vi "AA TCP Send Image.vi"(0 "Connection ID":refnum<k5>, 2 "Spooler Code":u8, 7 "Image Stack (U16)":u16[][][](array[numeric]), 11 "Error In":errorcluster, 13 "Setup Name":string) -> (4 "Connection ID Out":refnum<k5>, 8 "Success?":bool, 15 "Error Out":errorcluster)   [LabVIEW 2020]
panel:
  out "Image Size":i32[](array[numeric])
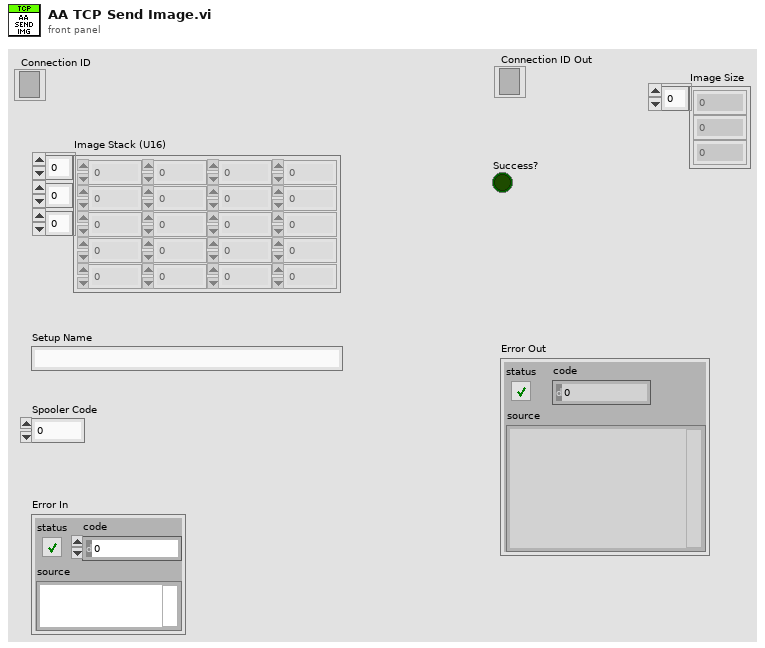
[diagram p1: front panel]
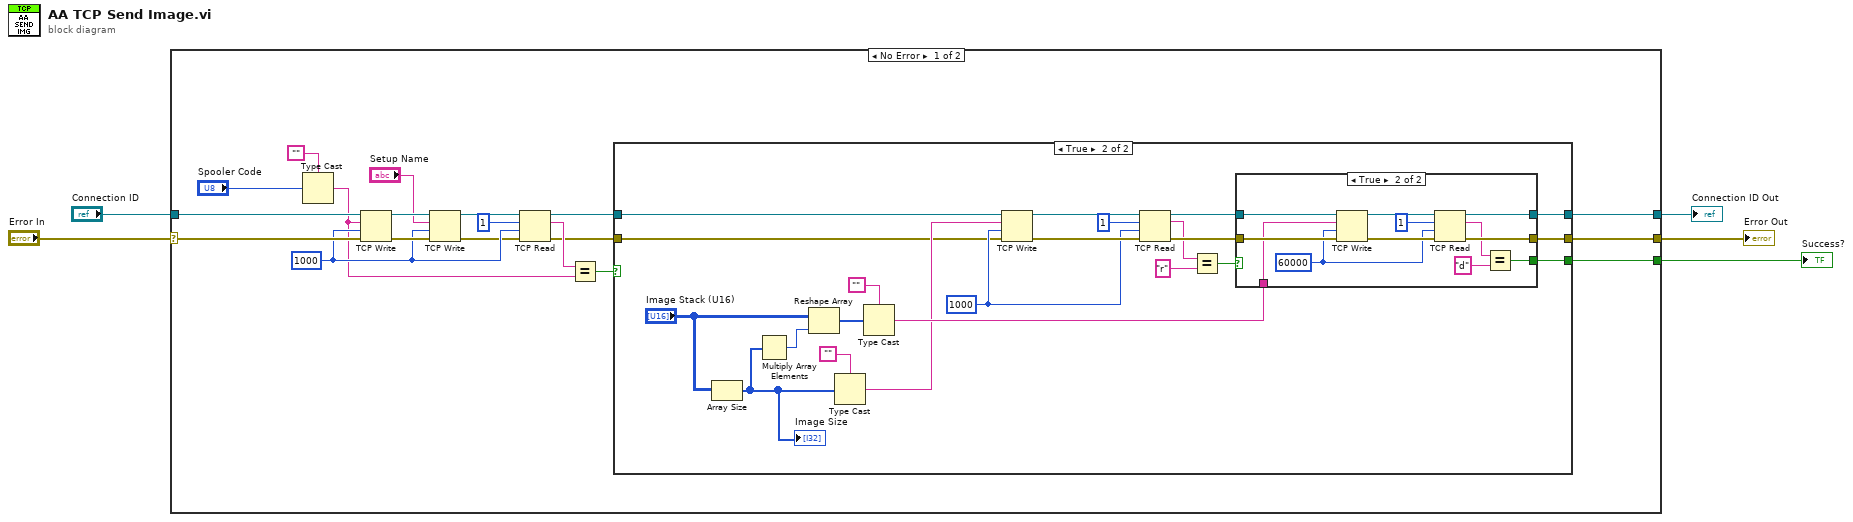
[diagram p0: block diagram]
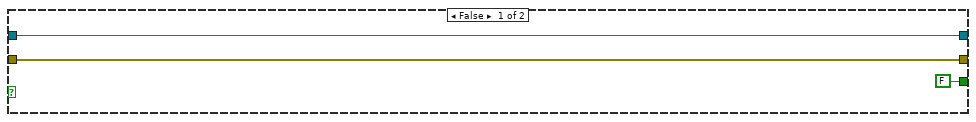
[diagram p2: hidden frame]
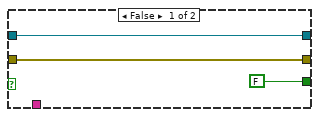
[diagram p3: hidden frame]
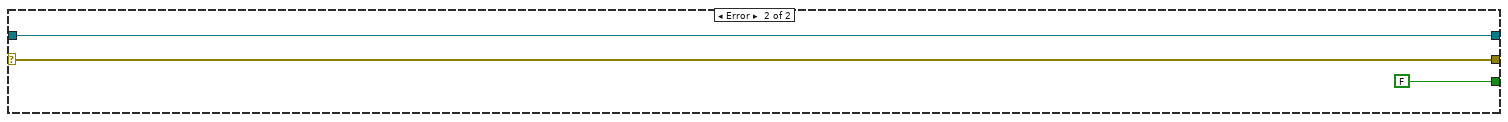
[diagram p4: hidden frame]
diagram:
  n1 = case shown="No Error" "Error In" {
    selector: "Error In" -> [w20 w66]
    tunnel: "Connection ID" -> [w21 w67]
    tunnel: [w24 w67] -> w4
    tunnel: [w23 w66] -> w3
    tunnel: [w22 FALSE] -> w2
    frame No Error {
      w11 = 1000 ("timeout ms (25000)")
      n2 = Type Cast(type="", x="Spooler Code") -> (*(type *) &x=w6:string)
      n3 = TCP Write(connection ID=w21, data in=w6, error in (no error)=w20, 9:w11) -> (connection ID out=w14:refnum<k5>, error out=w13:errorcluster)  [unwired: 1 out]
      n4 = TCP Write(connection ID=w14, data in="Setup Name", error in (no error)=w13, 9:w11) -> (connection ID out=w9:refnum<k5>, error out=w10:errorcluster)  [unwired: 1 out]
      n5 = TCP Read(connection ID=w9, bytes to read=1, error in (no error)=w10, 9:w11) -> (connection ID out=w16:refnum<k5>, data out=w19:string, error out=w15:errorcluster)  [unwired: 1 in]
      n6 = Equal?(x=w19, y=w6) -> (x = y?=w17:bool)
      n7 = case shown="True" w17 {
        tunnel: [w27 w45] -> w24
        tunnel: [w26 w40] -> w23
        tunnel: [FALSE w33] -> w22
        tunnel: w16 -> [w27 w29]
        tunnel: w15 -> [w26 w28]
        frame False {
        }
        frame True {
          w34 = 1000 ("timeout ms (25000)")
          n8 = Array Size(array="Image Stack (U16)") -> (size(s)=w32:i32[])
          "Image Size" <- w32
          n9 = Multiply Array Elements(1:w32) -> (0:w43:i32)
          n10 = Reshape Array("Image Stack (U16)", w43) -> (w49:u16[])
          n11 = Type Cast(type="", x=w32) -> (*(type *) &x=w31:string)
          n12 = Type Cast(type="", x=w49) -> (*(type *) &x=w35:string)
          n13 = TCP Write(connection ID=w29, data in=w31, error in (no error)=w28, 9:w34) -> (connection ID out=w47:refnum<k5>, error out=w42:errorcluster)  [unwired: 1 out]
          n14 = TCP Read(connection ID=w47, bytes to read=1, error in (no error)=w42, 9:w34) -> (connection ID out=w46:refnum<k5>, data out=w37:string, error out=w41:errorcluster)  [unwired: 1 in]
          n15 = Equal?(x=w37, y="r") -> (x = y?=w36:bool)
          n16 = case shown="True" w36 {
            tunnel: w46 -> [w52 w64]
            tunnel: [w52 w62] -> w45
            tunnel: w41 -> [w51 w61]
            tunnel: [w51 w59] -> w40
            tunnel: w35 -> [_ w58]
            tunnel: [FALSE w54] -> w33
            frame False {
            }
            frame True {
              w53 = 60000 ("timeout ms (25000)")
              n17 = TCP Write(connection ID=w64, data in=w58, error in (no error)=w61, 9:w53) -> (connection ID out=w63:refnum<k5>, error out=w60:errorcluster)  [unwired: 1 out]
              n18 = TCP Read(connection ID=w63, bytes to read=1, error in (no error)=w60, 9:w53) -> (connection ID out=w62:refnum<k5>, data out=w55:string, error out=w59:errorcluster)  [unwired: 1 in]
              n19 = Equal?(x=w55, y="d") -> (x = y?=w54:bool)
            }
          }
        }
      }
    }
    frame Error {
    }
  }
  "Connection ID Out" <- w4
  "Error Out" <- w3
  "Success?" <- w2
